vi "PNA_MAIN_RF_STATE.vi"(0 "Session In":refnum<visa-resource-name>="TCPIP0::K-Instr0000.local::inst0::INSTR", 11 "error in":errorcluster {"code" format="%.0x"}, 12 "RO(T)":bool, 14 "STATE(0=OFF)":i32(ring) items=["OFF", "ON"]) -> (3 "state(0 = off)":i8, 4 "Session Out":refnum<visa-resource-name>, 15 "error out":errorcluster {"code" format="%.0x"})   [LabVIEW 2018]
doc: "OUTPut[:STATe] <ON | OFF>\nApplicable Models: All\n\n(Read-Write) Turns RF power from the source ON or OFF."
panel:
  in  "Timeout":u32=3000
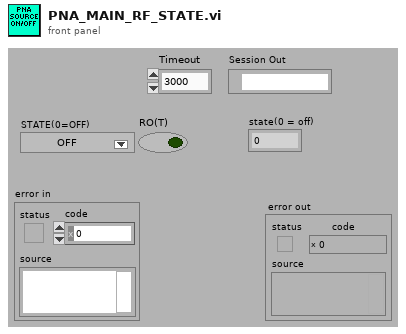
[diagram p1: front panel]
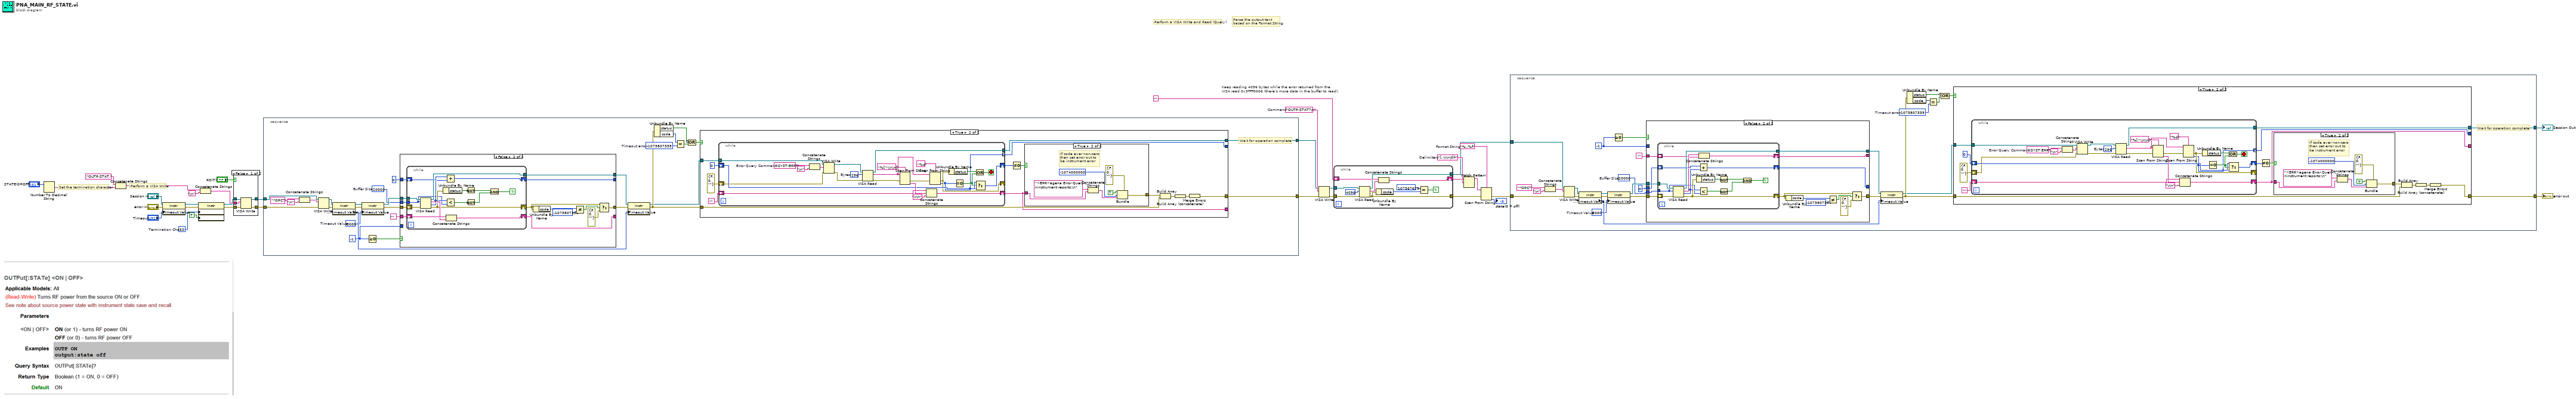
[diagram p0: block diagram]
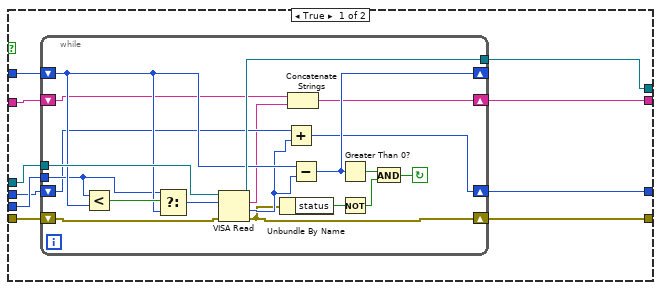
[diagram p2: hidden frame]
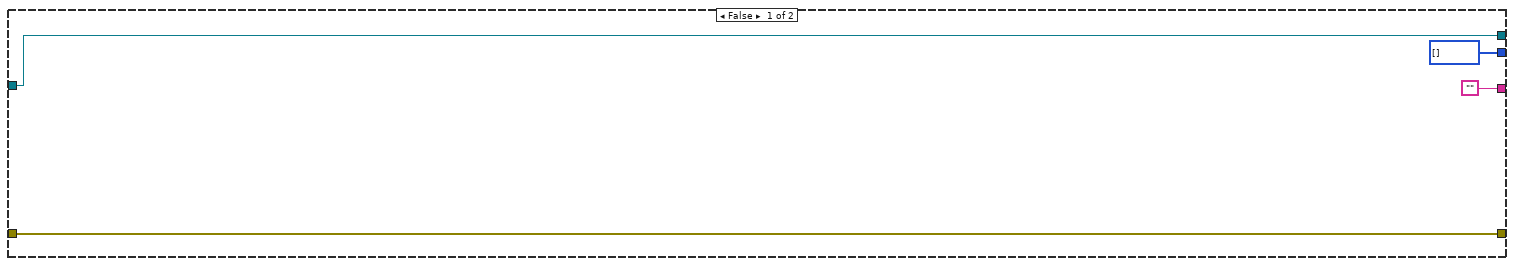
[diagram p3: hidden frame]
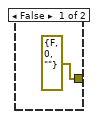
[diagram p4: hidden frame]
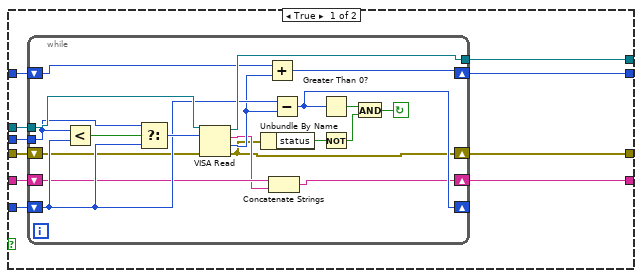
[diagram p5: hidden frame]
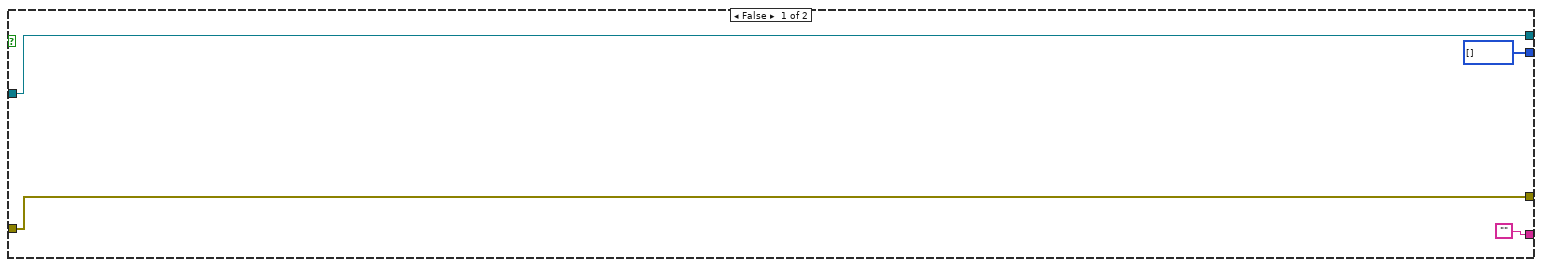
[diagram p6: hidden frame]
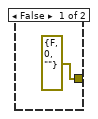
[diagram p7: hidden frame]
diagram:
  w11 = "[,;\r\n\t]+"  # Delimiters
  w13 = "%.;%f"  # Format String
  w16 = "OUTP:STAT?\n"  # Command
  w28 = u8 10  # Termination Char
  # "Parse the output text based on the Format String"
  # "Perform a VISA Write and Read (Query)"
  # "Keep reading 4096 bytes while the error returned from the\nVISA read 0x3FFF0006 (there's more data in the buffer to read)."
  # "Perform a VISA Write"
  # "Set the termination character"
  n1 = Number To Decimal String(number="STATE(0=OFF)") -> (decimal integer string=w25:string)  [unwired: 1 out]
  n2 = Concatenate Strings("OUTP:STAT " ("staticText"), w25) -> (w22:string)
  n3 = property class="Instr"(reference="Session In", error in="error in", "General Settings:Timeout Value"="Timeout") -> (reference out=w27:refnum<visa-resource-name>, error out=w30:errorcluster)
  n4 = property class="Instr"(reference=w27, error in=w30, "Message Based Settings:Termination Character"=w28, "Message Based Settings:Termination Character Enable"=TRUE ("enable")) -> (reference out=w10:refnum<visa-resource-name>, error out=w29:errorcluster)
  n5 = Concatenate Strings(w22, "\n" ("StaticText")) -> (w23:string)
  n6 = case shown="False" "RO(T)" {
    tunnel: w29 -> [w39 w40]
    tunnel: [w38 w40] -> w8
    tunnel: w23 -> [w37 _]
    tunnel: w10 -> [w36 w41]
    tunnel: [w35 w41] -> w7
    frame False {
      n7 = VISA Write(VISA resource name=w36, write buffer=w37, error in (no error)=w39) -> (VISA resource name out=w35:refnum<visa-resource-name>, error out=w38:errorcluster)  [unwired: 1 out]
    }
    frame True {
    }
  }
  n8 = stacked-sequence {
    tunnel: [w70] -> w5
    tunnel: [w69] -> w6
    tunnel: w8 -> [w63]
    tunnel: w7 -> [w61]
    frame #0 {
      w49 = u32 5000  # Timeout Value
      w45 = u32 20000  # Buffer Size
      w57 = -1073807339  # Timeout error
      w66 = -1 ("byte count")
      # "Wait for operation complete"
      n9 = Concatenate Strings("*OPC?" ("write buffer"), "\n") -> (w42:string)
      n10 = VISA Write(VISA resource name=w61, write buffer=w42, error in (no error)=w63) -> (VISA resource name out=w64:refnum<visa-resource-name>, error out=w65:errorcluster)  [unwired: 1 out]
      n11 = property class="Instr"(reference=w64, error in=w65) -> (reference out=w47:refnum<visa-resource-name>, error out=w48:errorcluster, "General Settings:Timeout Value"=w54:u32)
      n12 = property class="Instr"(reference=w47, error in=w48, "General Settings:Timeout Value"=w49) -> (reference out=w51:refnum<visa-resource-name>, error out=w50:errorcluster)
      n13 = Greater Or Equal To 0?(x=w66) -> (x >= 0?=w55:bool)
      n14 = case shown="False" w55 {
        tunnel: "" -> [w80 w113]
        tunnel: [w79 w112] -> _
        tunnel: w45 -> [w78 w111]
        tunnel: w66 -> [w77 _]
        tunnel: u32 0 ("byte count (0)") -> [w76 w110]
        tunnel: [w75 w109] -> _
        tunnel: w50 -> [w74 w108]
        tunnel: w51 -> [w73 w107]
        tunnel: [w72 w106] -> w52
        tunnel: [w71 w100] -> w53
        frame True {
          n15 = while {
            shift-left: w80 -> [w84]
            shift-right: [w85] -> w75
            tunnel: w78 -> [w93]
            shift-left: w76 -> [w91]
            shift-right: [w90] -> w79
            shift-left: w77 -> [w95]
            shift-right: [w94] -> _
            shift-left: w74 -> [w81]
            shift-right: [w82] -> w71
            tunnel: [w98] -> w72
            tunnel: w73 -> [w99]
            stop <- w86 continue-if-true
            n16 = Less?(x=w93, y=w95) -> (x < y?=w97:bool)
            n17 = Select(t=w93, s=w97, f=w95) -> (s? t:f=w96:u32)
            n18 = VISA Read(VISA resource name=w99, byte count=w96, error in (no error)=w81) -> (VISA resource name out=w98:refnum<visa-resource-name>, read buffer=w83:string, return count=w92:u32, error out=w82:errorcluster)
            n19 = Unbundle By Name(w82) -> ("status"=w88:bool)
            n20 = Add(x=w91, y=w92) -> (x+y=w90:u32)
            n21 = Concatenate Strings(w84, w83) -> (w85:string)
            n22 = Subtract(x=w95, y=w92) -> (x-y=w94:u32)
            n23 = Greater Than 0?(x=w94) -> (x > 0?=w89:bool)
            n24 = Not(x=w88) -> (.not. x?=w87:bool)
            n25 = And(x=w89, y=w87) -> (x .and. y?=w86:bool)
          }
        }
        frame False {
          n26 = while {
            shift-left: w113 -> [w123]
            shift-right: [w124] -> w109
            tunnel: w111 -> [w114]
            shift-left: w110 -> [w127]
            shift-right: [w126] -> w112
            shift-left: w108 -> [w120]
            shift-right: [w121] -> w102
            tunnel: [w128] -> w106
            tunnel: w107 -> [w129]
            stop <- w116 continue-if-true
            n27 = VISA Read(VISA resource name=w129, byte count=w114, error in (no error)=w120) -> (VISA resource name out=w128:refnum<visa-resource-name>, read buffer=w122:string, return count=w115:u32, error out=w121:errorcluster)
            n28 = Unbundle By Name(w121) -> ("status"=w125:bool)
            n29 = Add(x=w127, y=w115) -> (x+y=w126:u32)
            n30 = Less?(x=w115, y=w114) -> (x < y?=w119:bool)
            n31 = Concatenate Strings(w123, w122) -> (w124:string)
            n32 = Not(x=w125) -> (.not. x?=w117:bool)
            n33 = Not(x=w119) -> (.not. x?=w118:bool)
            n34 = And(x=w117, y=w118) -> (x .and. y?=w116:bool)
          }
          n35 = Unbundle By Name(w102) -> ("code"=w105:i32)
          n36 = Not Equal?(x=w105, y=-1073807339) -> (x != y?=w103:bool)
          n37 = Select(t=w102, s=w103, f=errorcluster {"status"=FALSE, "code"=0, "source"=""}) -> (s? t:f=w100:errorcluster)
        }
      }
      n38 = property class="Instr"(reference=w52, error in=w53, "General Settings:Timeout Value"=w54) -> (reference out=w67:refnum<visa-resource-name>, error out=w68:errorcluster)
      n39 = Unbundle By Name(w68) -> ("status"=w56:bool, "code"=w59:i32)
      n40 = Equal?(x=w59, y=w57) -> (x = y?=w58:bool)
      n41 = Compound Arithmetic op=OR(invert w56, w58) -> (w60:bool)
      n42 = case shown="True" w60 {
        tunnel: [w133 w147] -> w69
        tunnel: w67 -> [w133 w146]
        tunnel: w68 -> [w132 w140]
        tunnel: [w132 w144] -> w70
        tunnel: ["" w137] -> _
        tunnel: [i32[] [] w136] -> _
        frame False {
        }
        frame True {
          n43 = while {
            tunnel: [w180] -> w147
            tunnel: w146 -> [w179]
            shift-right: [w167] -> w137
            shift-left: "" -> [w170]
            shift-right: [w165] -> w138
            shift-left: 0 -> [w166]
            shift-right: [w163] -> _
            shift-left: errorcluster {"status"=FALSE, "code"=0, "source"=""} ("error in (no error)") -> [w164]
            tunnel: [w158] -> w136 mode=indexing
            stop <- w173 stop-if-true
            w177 = u32 256  # Bytes
            w175 = ":SYST:ERR?"  # Error Query Command
            n44 = Concatenate Strings(w175, "\n") -> (w156:string)
            n45 = VISA Write(VISA resource name=w179, write buffer=w156, error in (no error)=w164) -> (VISA resource name out=w178:refnum<visa-resource-name>, error out=w176:errorcluster)  [unwired: 1 out]
            n46 = VISA Read(VISA resource name=w178, byte count=w177, error in (no error)=w176) -> (VISA resource name out=w180:refnum<visa-resource-name>, read buffer=w171:string, error out=w162:errorcluster)  [unwired: 1 out]
            n47 = Scan From String(format string="%[^\\r\\n]", input string=w171, error in=w162) -> (error out=w161:errorcluster, output 1=w168:string)  [unwired: 2 in, 2 out]
            n48 = Concatenate Strings(w170, w168, "\r\n") -> (w167:string)
            n49 = Scan From String(format string="%d", input string=w171, error in=w161) -> (error out=w163:errorcluster, output 1=w158:i32)  [unwired: 2 in, 2 out]
            n50 = Unbundle By Name(w163) -> ("status"=w160:bool)
            n51 = Equal To 0?(x=w158) -> (x = 0?=w159:bool)
            n52 = Or(x=w160, y=w159) -> (x .or. y?=w173:bool)
            n53 = Select(t=w166, s=w159, f=w158) -> (s? t:f=w165:i32)
          }
          n54 = Not Equal To 0?(x=w138) -> (x != 0?=w142:bool)
          n55 = case shown="True" w142 {
            tunnel: w137 -> [_ w151]
            tunnel: [errorcluster {"status"=FALSE, "code"=0, "source"=""} ("error out") w150] -> w141
            frame False {
            }
            frame True {
              # "If code ever non-zero\nthen set error out to\nbe instrument error"
              n56 = Concatenate Strings("<ERR>agena Error Query;\ninstrument reports:\n" ("Source"), w151) -> (w152:string)
              n57 = Bundle(cluster=errorcluster {"status"=FALSE, "code"=0, "source"=""} ("error out"), "status"=TRUE ("Status"), "code"=-1074000000 ("Code"), "source"=w152) -> (w150:errorcluster)
            }
          }
          n58 = Build Array(w141, w140) -> (w135:errorcluster[])
          n59 = Build Array (concatenate)(w135) -> (w134:errorcluster[])
          n60 = Merge Errors(w134) -> (w144:errorcluster)
        }
      }
    }
  }
  n61 = VISA Write(VISA resource name=w6, write buffer=w16, error in (no error)=w5) -> (VISA resource name out=w20:refnum<visa-resource-name>, error out=w19:errorcluster)  [unwired: 1 out]
  n62 = while {
    tunnel: w20 -> [w188]
    shift-right: [w182] -> w15
    shift-left: "" -> [w187]
    tunnel: w19 -> [w185]
    tunnel: [w184] -> w18
    tunnel: [w181] -> w3
    stop <- w183 continue-if-true
    n63 = VISA Read(VISA resource name=w188, byte count=u32 4096 ("byte count (0)"), error in (no error)=w185) -> (VISA resource name out=w181:refnum<visa-resource-name>, read buffer=w186:string, error out=w184:errorcluster)  [unwired: 1 out]
    n64 = Unbundle By Name(w184) -> ("code"=w190:i32)
    n65 = Concatenate Strings(w187, w186) -> (w182:string)
    n66 = Equal?(x=1073676294, y=w190) -> (x = y?=w183:bool)
  }
  n67 = Match Pattern(string=w15, regular expression=w11) -> (before substring=w14:string)  [unwired: 1 in, 3 out]
  n68 = Scan From String(format string=w13, input string=w14, error in=w18) -> (error out=w4:errorcluster, output 1=→"state(0 = off)":i8)  [unwired: 2 in, 2 out]
  n69 = stacked-sequence {
    tunnel: [w220] -> w1
    tunnel: [w219] -> w2
    tunnel: w4 -> [w213]
    tunnel: w3 -> [w211]
    frame #0 {
      w199 = u32 5000  # Timeout Value
      w195 = u32 20000  # Buffer Size
      w207 = -1073807339  # Timeout error
      w216 = -1 ("byte count")
      # "Wait for operation complete"
      n70 = Concatenate Strings("*OPC?" ("write buffer"), "\n") -> (w192:string)
      n71 = VISA Write(VISA resource name=w211, write buffer=w192, error in (no error)=w213) -> (VISA resource name out=w214:refnum<visa-resource-name>, error out=w215:errorcluster)  [unwired: 1 out]
      n72 = property class="Instr"(reference=w214, error in=w215) -> (reference out=w197:refnum<visa-resource-name>, error out=w198:errorcluster, "General Settings:Timeout Value"=w204:u32)
      n73 = property class="Instr"(reference=w197, error in=w198, "General Settings:Timeout Value"=w199) -> (reference out=w201:refnum<visa-resource-name>, error out=w200:errorcluster)
      n74 = Greater Or Equal To 0?(x=w216) -> (x >= 0?=w205:bool)
      n75 = case shown="False" w205 {
        tunnel: "" -> [w230 w263]
        tunnel: [w229 w262] -> _
        tunnel: w195 -> [w228 w261]
        tunnel: w216 -> [w227 _]
        tunnel: u32 0 ("byte count (0)") -> [w226 w260]
        tunnel: [w225 w259] -> _
        tunnel: w200 -> [w224 w258]
        tunnel: w201 -> [w223 w257]
        tunnel: [w222 w256] -> w202
        tunnel: [w221 w250] -> w203
        frame True {
          n76 = while {
            shift-left: w230 -> [w234]
            shift-right: [w235] -> w225
            tunnel: w228 -> [w243]
            shift-left: w226 -> [w241]
            shift-right: [w240] -> w229
            shift-left: w227 -> [w245]
            shift-right: [w244] -> _
            shift-left: w224 -> [w231]
            shift-right: [w232] -> w221
            tunnel: [w248] -> w222
            tunnel: w223 -> [w249]
            stop <- w236 continue-if-true
            n77 = Less?(x=w243, y=w245) -> (x < y?=w247:bool)
            n78 = Select(t=w243, s=w247, f=w245) -> (s? t:f=w246:u32)
            n79 = VISA Read(VISA resource name=w249, byte count=w246, error in (no error)=w231) -> (VISA resource name out=w248:refnum<visa-resource-name>, read buffer=w233:string, return count=w242:u32, error out=w232:errorcluster)
            n80 = Unbundle By Name(w232) -> ("status"=w238:bool)
            n81 = Add(x=w241, y=w242) -> (x+y=w240:u32)
            n82 = Concatenate Strings(w234, w233) -> (w235:string)
            n83 = Subtract(x=w245, y=w242) -> (x-y=w244:u32)
            n84 = Greater Than 0?(x=w244) -> (x > 0?=w239:bool)
            n85 = Not(x=w238) -> (.not. x?=w237:bool)
            n86 = And(x=w239, y=w237) -> (x .and. y?=w236:bool)
          }
        }
        frame False {
          n87 = while {
            shift-left: w263 -> [w273]
            shift-right: [w274] -> w259
            tunnel: w261 -> [w264]
            shift-left: w260 -> [w277]
            shift-right: [w276] -> w262
            shift-left: w258 -> [w270]
            shift-right: [w271] -> w252
            tunnel: [w278] -> w256
            tunnel: w257 -> [w279]
            stop <- w266 continue-if-true
            n88 = VISA Read(VISA resource name=w279, byte count=w264, error in (no error)=w270) -> (VISA resource name out=w278:refnum<visa-resource-name>, read buffer=w272:string, return count=w265:u32, error out=w271:errorcluster)
            n89 = Unbundle By Name(w271) -> ("status"=w275:bool)
            n90 = Add(x=w277, y=w265) -> (x+y=w276:u32)
            n91 = Less?(x=w265, y=w264) -> (x < y?=w269:bool)
            n92 = Concatenate Strings(w273, w272) -> (w274:string)
            n93 = Not(x=w275) -> (.not. x?=w267:bool)
            n94 = Not(x=w269) -> (.not. x?=w268:bool)
            n95 = And(x=w267, y=w268) -> (x .and. y?=w266:bool)
          }
          n96 = Unbundle By Name(w252) -> ("code"=w255:i32)
          n97 = Not Equal?(x=w255, y=-1073807339) -> (x != y?=w253:bool)
          n98 = Select(t=w252, s=w253, f=errorcluster {"status"=FALSE, "code"=0, "source"=""}) -> (s? t:f=w250:errorcluster)
        }
      }
      n99 = property class="Instr"(reference=w202, error in=w203, "General Settings:Timeout Value"=w204) -> (reference out=w217:refnum<visa-resource-name>, error out=w218:errorcluster)
      n100 = Unbundle By Name(w218) -> ("status"=w206:bool, "code"=w209:i32)
      n101 = Equal?(x=w209, y=w207) -> (x = y?=w208:bool)
      n102 = Compound Arithmetic op=OR(invert w206, w208) -> (w210:bool)
      n103 = case shown="True" w210 {
        tunnel: [w283 w297] -> w219
        tunnel: w217 -> [w283 w296]
        tunnel: w218 -> [w282 w290]
        tunnel: [w282 w294] -> w220
        tunnel: ["" w287] -> _
        tunnel: [i32[] [] w286] -> _
        frame False {
        }
        frame True {
          n104 = while {
            tunnel: [w330] -> w297
            tunnel: w296 -> [w329]
            shift-right: [w317] -> w287
            shift-left: "" -> [w320]
            shift-right: [w315] -> w288
            shift-left: 0 -> [w316]
            shift-right: [w313] -> _
            shift-left: errorcluster {"status"=FALSE, "code"=0, "source"=""} ("error in (no error)") -> [w314]
            tunnel: [w308] -> w286 mode=indexing
            stop <- w323 stop-if-true
            w327 = u32 256  # Bytes
            w325 = ":SYST:ERR?"  # Error Query Command
            n105 = Concatenate Strings(w325, "\n") -> (w306:string)
            n106 = VISA Write(VISA resource name=w329, write buffer=w306, error in (no error)=w314) -> (VISA resource name out=w328:refnum<visa-resource-name>, error out=w326:errorcluster)  [unwired: 1 out]
            n107 = VISA Read(VISA resource name=w328, byte count=w327, error in (no error)=w326) -> (VISA resource name out=w330:refnum<visa-resource-name>, read buffer=w321:string, error out=w312:errorcluster)  [unwired: 1 out]
            n108 = Scan From String(format string="%[^\\r\\n]", input string=w321, error in=w312) -> (error out=w311:errorcluster, output 1=w318:string)  [unwired: 2 in, 2 out]
            n109 = Concatenate Strings(w320, w318, "\r\n") -> (w317:string)
            n110 = Scan From String(format string="%d", input string=w321, error in=w311) -> (error out=w313:errorcluster, output 1=w308:i32)  [unwired: 2 in, 2 out]
            n111 = Unbundle By Name(w313) -> ("status"=w310:bool)
            n112 = Equal To 0?(x=w308) -> (x = 0?=w309:bool)
            n113 = Or(x=w310, y=w309) -> (x .or. y?=w323:bool)
            n114 = Select(t=w316, s=w309, f=w308) -> (s? t:f=w315:i32)
          }
          n115 = Not Equal To 0?(x=w288) -> (x != 0?=w292:bool)
          n116 = case shown="True" w292 {
            tunnel: w287 -> [_ w301]
            tunnel: [errorcluster {"status"=FALSE, "code"=0, "source"=""} ("error out") w300] -> w291
            frame False {
            }
            frame True {
              # "If code ever non-zero\nthen set error out to\nbe instrument error"
              n117 = Concatenate Strings("<ERR>agena Error Query;\ninstrument reports:\n" ("Source"), w301) -> (w302:string)
              n118 = Bundle(cluster=errorcluster {"status"=FALSE, "code"=0, "source"=""} ("error out"), "status"=TRUE ("Status"), "code"=-1074000000 ("Code"), "source"=w302) -> (w300:errorcluster)
            }
          }
          n119 = Build Array(w291, w290) -> (w285:errorcluster[])
          n120 = Build Array (concatenate)(w285) -> (w284:errorcluster[])
          n121 = Merge Errors(w284) -> (w294:errorcluster)
        }
      }
    }
  }
  "error out" <- w1
  "Session Out" <- w2
